vi "week2_graphs-vs-charts_LV18.vi"() -> ()   [LabVIEW 2018]
uses:
  <vilib>/numeric/Random Number (Range) U64.vi
panel:
  out "Raw Data Array":dbl[](array[numeric])=[0.0, 0.0, 0.0, 0.0, 0.0, 0.0, 0.0, 0.0, 0.0, 0.0, 677.0, 681.0, 661.0, 695.0, 692.0, 690.0, 629.0, 709.0, 748.0, 772.0, 819.0, 885.0, 949.0, 1054.0, 1162.0, 1315.0, 1476.0, 1662.0, 1873.0, 2071.0, 2250.0, 2431.0, 2570.0, 2674.0, 2745.0, 2777.0, 2821.0, 2825.0, 2867.0, 2884.0, 2906.0, 2967.0, 3016.0, 3097.0, 3214.0, 3339.0, 3499.0, 3682.0, 3909.0, 4147.0, 4406.0, 4693.0, 4985.0, 5268.0, 5531.0, 5752.0, 5957.0, 6073.0, 6134.0, 6119.0, 6036.0, 5913.0, 5725.0, 5521.0, 5307.0, 5107.0, 4909.0, 4724.0, 4564.0, 4422.0, 4315.0, 4236.0, 4168.0, 4115.0, 4100.0, 4105.0, 4108.0, 4125.0, 4187.0, 4254.0, 4321.0, 4421.0, 4535.0, 4672.0, 4821.0, 4965.0, 5119.0, 5267.0, 5394.0, 5499.0, 5586.0, 5656.0, 5683.0, 5652.0, 5605.0, 5502.0, 5403.0, 5257.0, 5095.0, 4943.0, 4756.0, 4601.0, 4418.0, 4305.0, 4176.0, 4049.0, 3950.0, 3875.0, 3815.0, 3764.0, 3741.0, 3718.0, 3703.0, 3696.0, 3741.0, 3777.0, 3826.0, 3891.0, 3973.0, 4068.0, 4184.0, 4293.0, 4417.0, 4578.0, 4733.0, 4909.0, 5097.0, 5268.0, 5467.0, 5655.0, 5816.0, 6021.0, 6184.0, 6322.0, 6464.0, 6542.0, 6613.0, 6668.0, 6684.0, 6672.0, 6623.0, 6587.0, 6498.0, 6409.0, 6301.0, 6136.0, 6043.0, 5924.0, 5768.0, 5659.0, 5517.0, 5401.0, 5281.0, 5154.0, 5070.0, 4980.0, 4902.0, 4823.0, 4774.0, 4709.0, 4649.0, 4618.0, 4598.0, 4566.0, 4537.0, 4533.0, 4519.0, 4500.0, 4496.0, 4490.0, 4480.0, 4485.0, 4492.0, 4487.0, 4512.0, 4530.0, 4556.0, 4598.0, 4638.0, 4689.0, 4734.0, 4783.0, 4822.0, 4850.0, 4907.0, 4926.0, 4962.0, 4988.0, 4965.0, 5050.0, 5050.0, 5079.0, 5069.0, 5077.0, 5063.0, 5057.0, 5063.0, 5043.0, 5019.0, 4992.0, 4968.0, 4932.0, 4884.0, 4821.0, 4762.0, 4694.0, 4626.0, 4547.0, 4467.0, 4389.0, 4317.0, 4232.0, 4151.0, 4054.0, 3985.0, 3912.0, 3848.0, 3809.0, 3733.0, 3666.0, 3593.0, 3518.0, 3459.0, 3401.0, 3355.0, 3319.0, 3284.0, 3263.0, 3251.0, 3242.0, 3232.0, 3195.0, 3229.0, 3220.0, 3184.0, 3163.0, 3155.0, 3152.0, 3136.0, 3132.0, 3098.0, 3115.0, 3127.0, 3129.0, 3124.0, 3117.0, 3140.0, 3194.0, 3225.0, 3237.0, 3217.0, 3121.0, 3013.0, 2864.0, 2722.0, 2475.0]
  out "Waveform Graph 2":dynamicdata(graph)
  out "XY Graph":cluster{"Y":dbl[], "Y":dbl[]}[](graph)
  out "Waveform Graph":u64[](graph)
  out "Waveform Chart":u64(graph)
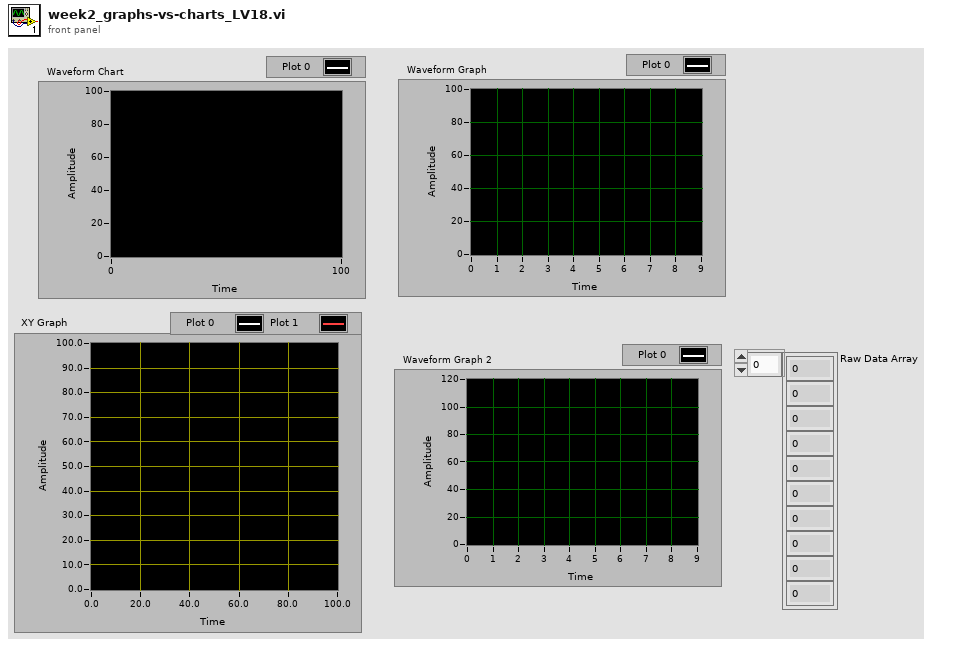
[diagram p1: front panel]
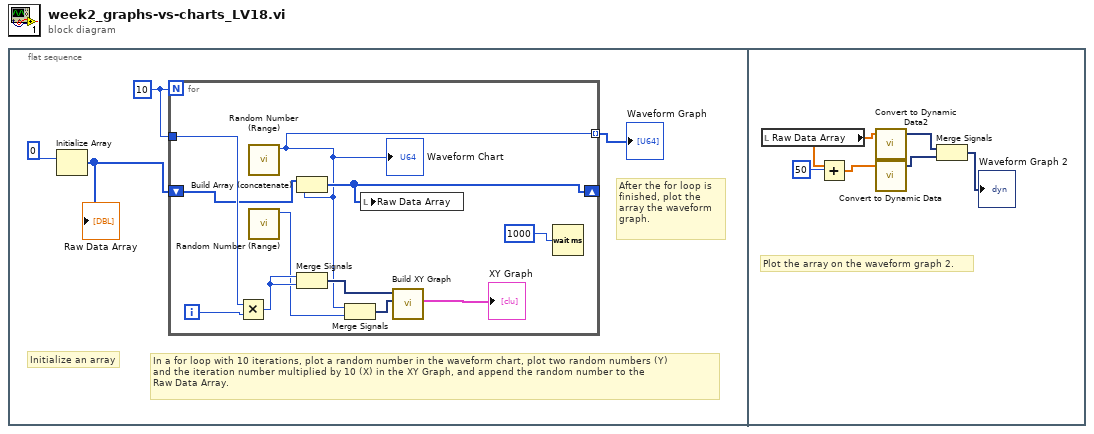
[diagram p0: block diagram]
diagram:
  n1 = flat-sequence {
    frame #0 {
      w3 = 10
      # "After the for loop is \nfinished, plot the \narray the waveform\ngraph."
      # "In a for loop with 10 iterations, plot a random number in the waveform chart, plot two random numbers (Y)\nand the iteration number multiplied by 10 (X) in the XY Graph, and append the random number to the \nRaw Data Array."
      # "Initialize an array"
      n2 = Initialize Array(0) -> (w1:i32[])  [unwired: 1 in]
      "Raw Data Array" <- w1
      n3 = for {
        N: w3 -> [_]
        tunnel: w3 -> [w14]
        tunnel: [w6] -> w4 mode=indexing
        shift-right: [w12] -> _
        shift-left: w1 -> [w11]
        i -> [w9]
        n4 = Multiply(x=w14, y=w9) -> (x*y=w8:i32)
        n5 = call-poly <vilib>:"Random Number (Range).vi"() -> ("number"=w6:u64)  [unwired: 11 in]
        "Waveform Chart" <- w6
        n6 = call-poly <vilib>:"Random Number (Range).vi"() -> ("number"=w7:u64)  [unwired: 11 in]
        n7 = Build Array (concatenate)(w11, w6) -> (w12:u64[])
        n8 = Merge Signals(w8, w8) -> (w10:dynamicdata)
        n9 = Merge Signals(w6, w7) -> (w5:dynamicdata)
        n10 = local write "Raw Data Array"(w12) -> ()
        n11 = call "Build XY Graph"("Y Input"=w5, "X Input"=w10) -> ("XY Graph"=→"XY Graph":cluster{"X":dbl[], "Y":dbl[]}[])  [unwired: 8 in, 1 out]
        n12 = Wait (ms)(milliseconds to wait=1000) -> ()  [unwired: 1 out]
      }
      "Waveform Graph" <- w4
    }
    frame #1 {
      # "Plot the array on the waveform graph 2."
      n13 = local read "Raw Data Array"() -> (w18:dbl[])
      n14 = Add(x=w18, y=50) -> (x+y=w20:dbl[])
      n15 = call "Convert to Dynamic Data2"("Array"=w18) -> ("Dynamic Data Type"=w17:dynamicdata)  [unwired: 3 in]
      n16 = call "Convert to Dynamic Data"("Array"=w20) -> ("Dynamic Data Type"=w19:dynamicdata)  [unwired: 3 in]
      n17 = Merge Signals(w17, w19) -> (→"Waveform Graph 2":dynamicdata)
    }
  }
